vi "Table Select All.vi"(11 "Table Ref In":refnum<vi>) -> (3 "Table Ref Out":refnum<vi>)   [LabVIEW 2024]
uses:
  <vilib>/Utility/miscctls.llb/LVRowAndColumnTypeDef.ctl
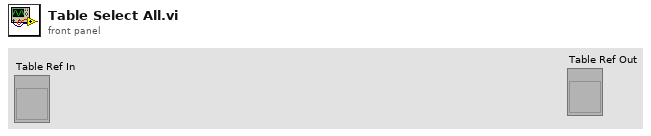
[diagram p1: front panel]
types:
  T1 = typedef "LVRowAndColumnTypeDef.ctl" = cluster{"Row":i32, "Column":i32}
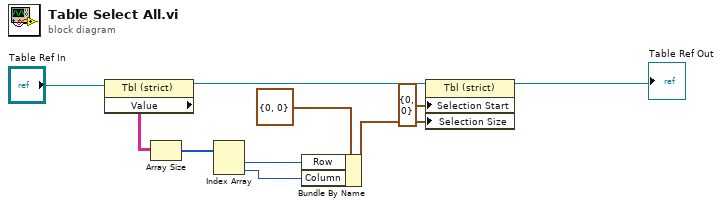
[diagram p0: block diagram]
diagram:
  n1 = property class="Tbl (strict)"(reference="Table Ref In") -> (reference out=w9:refnum<vi>, "Value"=w7:string[][])  [unwired: 1 in, 1 out]
  n2 = Array Size(array=w7) -> (size(s)=w5:i32[])
  n3 = Index Array(array=w5) -> (element #1=w3:i32, element #2=w2:i32)  [unwired: 2 in]
  n4 = Bundle By Name(cluster=T1 {"Row"=0, "Column"=0} ("Selection Size"), "Row"=w3, "Column"=w2) -> (w1:T1)
  n5 = property class="Tbl (strict)"(reference=w9, "Selection Start"=T1 {"Row"=0, "Column"=0}, "Selection Size"=w1) -> (reference out=→"Table Ref Out":refnum<vi>)  [unwired: 1 in, 1 out]
